vi "AcquireImage(Cont).vi"(8 "error in (no error)":errorcluster, 10 "timeout (s)":dbl=1.0 format="%#_13g", 11 "CameraSession in":refnum<class "CS250-CameraHardwareClass.lvclass">) -> (0 "error out":errorcluster, 2 "ready":bool, 3 "CameraSession out":refnum<class "CS250-CameraHardwareClass.lvclass">)   [LabVIEW 2013, in "CS250-CameraHardwareClass.lvclass"]
uses:
  CS250-CameraHardwareClass.lvclass
  CS250-CameraHardwareClass.lvclass/CS250-CameraHardwareClass.ctl
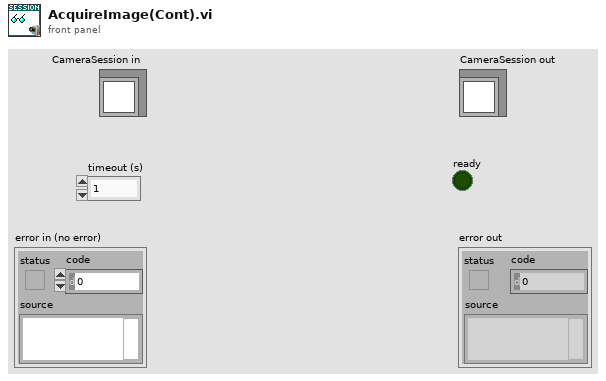
[diagram p1: front panel]
types:
  T1 = typedef "CamCluster.ctl" = cluster{"hcam out":i16, "TempImage":T2, "Pointer":u32, "exp_bytes out":u32, "rgn_array":cluster{"s1":u16, "s2":u16, "sbin":u16, "p1":u16, "p2":u16, "pbin":u16}, "CameraName":string}
  T2 = typedef "IMAQ Image.ctl" = refnum<image>
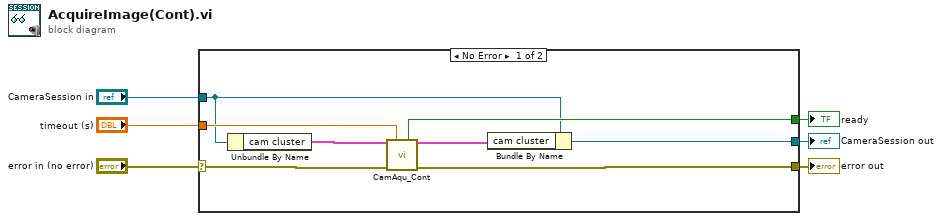
[diagram p0: block diagram]
diagram:
  n1 = case shown="No Error" "error in (no error)" {
    selector: "error in (no error)" -> [w12 w16]
    tunnel: [w11 w16] -> w5
    tunnel: [w7 w15] -> w3
    tunnel: "CameraSession in" -> [w9 w15]
    tunnel: "timeout (s)" -> [w13 _]
    tunnel: [w10 _] -> w1
    frame No Error {
      n2 = Unbundle By Name(w9) -> ("cam cluster"=w14:T1)
      n3 = call "CamAqu_Cont.vi"("cam cluster in"=w14, "timeout (s)"=w13, "error in (no error)"=w12) -> ("ready"=w10:bool, "cam cluster out"=w8:T1, "error out"=w11:errorcluster)  [unwired: 10 in]
      n4 = Bundle By Name(cluster=w9, "cam cluster"=w8) -> (w7:refnum<class "CS250-CameraHardwareClass.lvclass">)
    }
    frame Error {
    }
  }
  "error out" <- w5
  "CameraSession out" <- w3
  "ready" <- w1
